vi "S4GUI_003.vi"(7 "Tab ObsEng":enum32{"Obs", "CCD modes", "Guider", "Eng"}(tab)) -> ()   [LabVIEW 2018] (continued)
        n4627 = call "Read WPROT.vi"("error in (no error)"=w10973, "Instrument in"=w10974) -> ("error out"=w10969:errorcluster, "Opt_Selector.lvclass"=w10972:refnum<class "Opt_Selector.lvclass">, "Instrument out"=w10965:refnum<class "Instrument.lvclass">)  [unwired: 7 in]
        n4628 = call-dynamic "Read State Machine.vi"("error in (no error)"=w10969, "Device in"=w10972) -> ("error out"=w10968:errorcluster, "State Machine.lvclass"=w10971:refnum<class "State Machine.lvclass">, "Device out"=w10967:refnum<class "Opt_Selector.lvclass">)  [unwired: 7 in]
        n4629 = call "Next State.vi"("error in (no error)"=w10968, "New_State"=1, "State Machine in"=w10971) -> ("error out"=w10956:errorcluster, "State Machine out"=w10958:refnum<class "State Machine.lvclass">)  [unwired: 7 in]
        n4630 = call-dynamic "Write Timer.vi"("error in (no error)"=w10956, "Timer"=u32 10, "State Machine in"=w10958) -> ("error out"=w10955:errorcluster, "State Machine out"=w10957:refnum<class "State Machine.lvclass">)  [unwired: 7 in]
        n4631 = call-dynamic "Write State Machine.vi"("error in (no error)"=w10955, "State Machine.lvclass"=w10957, "Device in"=w10967) -> ("error out"=w10964:errorcluster, "Device out"=w10966:refnum<class "Opt_Selector.lvclass">)  [unwired: 7 in]
        n4632 = call "Write WPROT.vi"("error in (no error)"=w10964, "Opt_Selector.lvclass"=w10966, "Instrument in"=w10965) -> ("error out"=w10961:errorcluster, "Instrument out"=w10963:refnum<class "Instrument.lvclass">)  [unwired: 7 in]
        n4633 = call "Write Instrument.lvclass.vi"("error in (no error)"=w10961, "Instrument.lvclass"=w10963, "S4ACS_GUI in"=w10962) -> ("error out"=w10960:errorcluster, "S4ACS_GUI out"=w10959:refnum<class "S4GUI.lvclass">)  [unwired: 7 in]
      }
      event "TARGET NAME WPROT": Value Change {
        n4634 = event-data() -> ()  [unwired: 1 in, 1 out]
        n4635 = call "Read Instrument.lvclass.vi"("error in (no error)"=w11004, "S4ACS_GUI in"=w11005) -> ("error out"=w11012:errorcluster, "Instrument.lvclass"=w11013:refnum<class "Instrument.lvclass">, "S4ACS_GUI out"=w11007:refnum<class "S4GUI.lvclass">)  [unwired: 7 in]
        n4636 = property on="TARGET NAME WPROT" class="Enum (strict)"() -> ("RingText.Text"=w11003:string)  [unwired: 2 in, 2 out]
        n4637 = Build Array(-1.0 ("element"), 0.0 ("element"), 22.5 ("element"), 45.0 ("element"), 67.5 ("element"), 90.0 ("element"), 112.5 ("element"), 135.0 ("element"), 157.5 ("element"), 180.0 ("element"), 202.5 ("element"), 225.0 ("element"), 247.5 ("element"), 270.0 ("element"), 292.5 ("element"), 315.0 ("element"), 337.5 ("element")) -> (w10995:dbl[])
        n4638 = call "Read WPROT.vi"("error in (no error)"=w11012, "Instrument in"=w11013) -> ("error out"=w11010:errorcluster, "Opt_Selector.lvclass"=w11011:refnum<class "Opt_Selector.lvclass">, "Instrument out"=w11009:refnum<class "Instrument.lvclass">)  [unwired: 7 in]
        n4639 = call "Write target name.vi"("error in (no error)"=w11010, "target name"=w11003, "Optics in"=w11011) -> ("error out"=w10991:errorcluster, "Optics out"=w10992:refnum<class "Opt_Selector.lvclass">)  [unwired: 7 in]
        n4640 = Index Array(array=w10995, index="TARGET NAME WPROT") -> (element=w10993:dbl)
        n4641 = call "Write target.vi"("error in (no error)"=w10991, "target"=w10993, "Optics in"=w10992) -> ("error out"=w10990:errorcluster, "Optics out"=w10989:refnum<class "Opt_Selector.lvclass">)  [unwired: 7 in]
        n4642 = call "Write WPROT.vi"("error in (no error)"=w10990, "Opt_Selector.lvclass"=w10989, "Instrument in"=w11009) -> ("error out"=w11006:errorcluster, "Instrument out"=w11008:refnum<class "Instrument.lvclass">)  [unwired: 7 in]
        n4643 = call "Write Instrument.lvclass.vi"("error in (no error)"=w11006, "Instrument.lvclass"=w11008, "S4ACS_GUI in"=w11007) -> ("error out"=w11002:errorcluster, "S4ACS_GUI out"=w10977:refnum<class "S4GUI.lvclass">)  [unwired: 7 in]
      }
      event "TARGET NAME WPSEL": Value Change {
        n4644 = event-data() -> ()  [unwired: 1 in, 1 out]
        n4645 = call "Read Instrument.lvclass.vi"("error in (no error)"=w11028, "S4ACS_GUI in"=w11029) -> ("error out"=w11036:errorcluster, "Instrument.lvclass"=w11037:refnum<class "Instrument.lvclass">, "S4ACS_GUI out"=w11031:refnum<class "S4GUI.lvclass">)  [unwired: 7 in]
        n4646 = property on="TARGET NAME WPSEL" class="Enum (strict)"() -> ("RingText.Text"=w11015:string)  [unwired: 2 in, 2 out]
        n4647 = Build Array(-1.0 ("element"), 80.0 ("element"), 0.0 ("element"), 160.0 ("element")) -> (w11022:dbl[])
        n4648 = call "Read WPSEL.vi"("error in (no error)"=w11036, "Instrument in"=w11037) -> ("error out"=w11034:errorcluster, "Opt_Selector.lvclass"=w11035:refnum<class "Opt_Selector.lvclass">, "Instrument out"=w11033:refnum<class "Instrument.lvclass">)  [unwired: 7 in]
        n4649 = call "Write target name.vi"("error in (no error)"=w11034, "target name"=w11015, "Optics in"=w11035) -> ("error out"=w11019:errorcluster, "Optics out"=w11020:refnum<class "Opt_Selector.lvclass">)  [unwired: 7 in]
        n4650 = Index Array(array=w11022, index="TARGET NAME WPSEL") -> (element=w11021:dbl)
        n4651 = call "Write target.vi"("error in (no error)"=w11019, "target"=w11021, "Optics in"=w11020) -> ("error out"=w11018:errorcluster, "Optics out"=w11017:refnum<class "Opt_Selector.lvclass">)  [unwired: 7 in]
        n4652 = call "Write WPSEL.vi"("error in (no error)"=w11018, "Opt_Selector.lvclass"=w11017, "Instrument in"=w11033) -> ("error out"=w11030:errorcluster, "Instrument out"=w11032:refnum<class "Instrument.lvclass">)  [unwired: 7 in]
        n4653 = call "Write Instrument.lvclass.vi"("error in (no error)"=w11030, "Instrument.lvclass"=w11032, "S4ACS_GUI in"=w11031) -> ("error out"=w11027:errorcluster, "S4ACS_GUI out"=w11014:refnum<class "S4GUI.lvclass">)  [unwired: 7 in]
      }
      event "Lambda Selector": Value Change {
        n4654 = event-data() -> ("NewVal"=w11039:u16)  [unwired: 1 in, 1 out]
        n4655 = call "Read Instrument.lvclass.vi"("error in (no error)"=w11070, "S4ACS_GUI in"=w11071) -> ("error out"=w11072:errorcluster, "Instrument.lvclass"=w11047:refnum<class "Instrument.lvclass">, "S4ACS_GUI out"=w11044:refnum<class "S4GUI.lvclass">)  [unwired: 7 in]
        n4656 = Build Array(80.0 ("element"), 0.0 ("element"), 160.0 ("element")) -> (w11065:dbl[])
        n4657 = property on="Lambda Selector" class="Ring (strict)"() -> ("RingText.Text"=w11045:string)  [unwired: 2 in, 2 out]
        n4658 = call "Read WPSEL.vi"("error in (no error)"=w11072, "Instrument in"=w11047) -> ("error out"=w11054:errorcluster, "Opt_Selector.lvclass"=w11053:refnum<class "Opt_Selector.lvclass">, "Instrument out"=w11046:refnum<class "Instrument.lvclass">)  [unwired: 7 in]
        n4659 = Index Array(array=w11065, index=w11039) -> (element=w11064:dbl)
        n4660 = call "Write target.vi"("error in (no error)"=w11054, "target"=w11064, "Optics in"=w11053) -> ("error out"=w11051:errorcluster, "Optics out"=w11052:refnum<class "Opt_Selector.lvclass">)  [unwired: 7 in]
        n4661 = case shown="\"OFF\", Default" w11045 {
          selector: w11045 -> [w11075 _ _]
          tunnel: [w11075 "ON" "ON"] -> w11056
          tunnel: [0.0 ("element") 30.0 ("element") 30.0 ("element")] -> w11055
          tunnel: [w11075 "L/2" "L/4"] -> w11048
          frame "OFF", Default {
            n4662 = property on="Calibrator Selector" class="Ring (strict)"("DisabledEnum"=T12."Disabled and Grayed Out" ("Disabled")) -> ()  [unwired: 2 in, 2 out]
          }
          frame "Lambda/2" {
            n4663 = property on="Calibrator Selector" class="Ring (strict)"("DisabledEnum"=T12."Enabled" ("Disabled")) -> ()  [unwired: 2 in, 2 out]
          }
          frame "Lambda/4" {
            n4664 = property on="Calibrator Selector" class="Ring (strict)"("DisabledEnum"=T12."Enabled" ("Disabled")) -> ()  [unwired: 2 in, 2 out]
          }
        }
        n4665 = call "Write target name.vi"("error in (no error)"=w11051, "target name"=w11048, "Optics in"=w11052) -> ("error out"=w11050:errorcluster, "Optics out"=w11049:refnum<class "Opt_Selector.lvclass">)  [unwired: 7 in]
        n4666 = call "Write WPSEL.vi"("error in (no error)"=w11050, "Opt_Selector.lvclass"=w11049, "Instrument in"=w11046) -> ("error out"=w11041:errorcluster, "Instrument out"=w11040:refnum<class "Instrument.lvclass">)  [unwired: 7 in]
        n4667 = call "Read ASEL.vi"("error in (no error)"=w11041, "Instrument in"=w11040) -> ("error out"=w11061:errorcluster, "Opt_Selector.lvclass"=w11059:refnum<class "Opt_Selector.lvclass">, "Instrument out"=w11043:refnum<class "Instrument.lvclass">)  [unwired: 7 in]
        n4668 = call "Write target name.vi"("error in (no error)"=w11061, "target name"=w11056, "Optics in"=w11059) -> ("error out"=w11062:errorcluster, "Optics out"=w11058:refnum<class "Opt_Selector.lvclass">)  [unwired: 7 in]
        n4669 = call "Write target.vi"("error in (no error)"=w11062, "target"=w11055, "Optics in"=w11058) -> ("error out"=w11063:errorcluster, "Optics out"=w11057:refnum<class "Opt_Selector.lvclass">)  [unwired: 7 in]
        n4670 = call "Write ASEL.vi"("error in (no error)"=w11063, "Opt_Selector.lvclass"=w11057, "Instrument in"=w11043) -> ("error out"=w11060:errorcluster, "Instrument out"=w11042:refnum<class "Instrument.lvclass">)  [unwired: 7 in]
        n4671 = call "Write Instrument.lvclass.vi"("error in (no error)"=w11060, "Instrument.lvclass"=w11042, "S4ACS_GUI in"=w11044) -> ("error out"=w11069:errorcluster, "S4ACS_GUI out"=w11038:refnum<class "S4GUI.lvclass">)  [unwired: 7 in]
      }
      event "Calibrator Selector": Value Change {
        n4672 = event-data() -> ()  [unwired: 1 in, 6 out]
        n4673 = call "Read Instrument.lvclass.vi"("error in (no error)"=w11104, "S4ACS_GUI in"=w11105) -> ("error out"=w11108:errorcluster, "Instrument.lvclass"=w11109:refnum<class "Instrument.lvclass">, "S4ACS_GUI out"=w11106:refnum<class "S4GUI.lvclass">)  [unwired: 7 in]
        n4674 = Build Array(0.0 ("element"), 72.0 ("element"), 144.0 ("element"), 216.0 ("element"), 288.0 ("element")) -> (w11099:dbl[])
        n4675 = call "Read CALW.vi"("error in (no error)"=w11108, "Instrument in"=w11109) -> ("error out"=w11097:errorcluster, "Opt_Selector.lvclass"=w11096:refnum<class "Opt_Selector.lvclass">, "Instrument out"=w11107:refnum<class "Instrument.lvclass">)  [unwired: 7 in]
        n4676 = Index Array(array=w11099, index="Calibrator Selector") -> (element=w11098:dbl)
        n4677 = call "Write target.vi"("error in (no error)"=w11097, "target"=w11098, "Optics in"=w11096) -> ("error out"=w11094:errorcluster, "Optics out"=w11095:refnum<class "Opt_Selector.lvclass">)  [unwired: 7 in]
        n4678 = property on="Calibrator Selector" class="Ring (strict)"() -> ("RingText.Text"=w11090:string)  [unwired: 2 in, 2 out]
        n4679 = case shown="\"POLARIZER\"" w11090 {
          selector: w11090 -> [_ w11111 w11112 w11113 w11114]
          tunnel: ["OFF" w11111 w11112 w11113 w11114] -> w11091
          frame "OFF", Default {
          }
          frame "POLARIZER" {
          }
          frame "DEPOLARIZER" {
          }
          frame "PINHOLE" {
          }
          frame "SHUTTER" {
          }
        }
        n4680 = call "Write target name.vi"("error in (no error)"=w11094, "target name"=w11091, "Optics in"=w11095) -> ("error out"=w11093:errorcluster, "Optics out"=w11092:refnum<class "Opt_Selector.lvclass">)  [unwired: 7 in]
        n4681 = call "Write CALW.vi"("error in (no error)"=w11093, "Opt_Selector.lvclass"=w11092, "Instrument in"=w11107) -> ("error out"=w11087:errorcluster, "Instrument out"=w11088:refnum<class "Instrument.lvclass">)  [unwired: 7 in]
        n4682 = call "Write Instrument.lvclass.vi"("error in (no error)"=w11087, "Instrument.lvclass"=w11088, "S4ACS_GUI in"=w11106) -> ("error out"=w11103:errorcluster, "S4ACS_GUI out"=w11086:refnum<class "S4GUI.lvclass">)  [unwired: 7 in]
      }
      event "TARGET NAME CALW": Value Change {
        # "aqui também"
        # "OV20230825: Valores da sequência original"
        n4683 = event-data() -> ()  [unwired: 1 in, 6 out]
        n4684 = call "Read Instrument.lvclass.vi"("error in (no error)"=w11131, "S4ACS_GUI in"=w11132) -> ("error out"=w11139:errorcluster, "Instrument.lvclass"=w11140:refnum<class "Instrument.lvclass">, "S4ACS_GUI out"=w11134:refnum<class "S4GUI.lvclass">)  [unwired: 7 in]
        n4685 = property on="TARGET NAME CALW" class="Enum (strict)"() -> ("RingText.Text"=w11115:string)  [unwired: 2 in, 2 out]
        n4686 = Build Array(-1.0 ("element"), 0.0 ("element"), 72.0 ("element"), 144.0 ("element"), 216.0 ("element"), 288.0 ("element")) -> (w11125:dbl[])
        n4687 = call "Read CALW.vi"("error in (no error)"=w11139, "Instrument in"=w11140) -> ("error out"=w11137:errorcluster, "Opt_Selector.lvclass"=w11138:refnum<class "Opt_Selector.lvclass">, "Instrument out"=w11136:refnum<class "Instrument.lvclass">)  [unwired: 7 in]
        n4688 = call "Write target name.vi"("error in (no error)"=w11137, "target name"=w11115, "Optics in"=w11138) -> ("error out"=w11122:errorcluster, "Optics out"=w11123:refnum<class "Opt_Selector.lvclass">)  [unwired: 7 in]
        n4689 = Index Array(array=w11125, index="TARGET NAME CALW") -> (element=w11124:dbl)
        n4690 = call "Write target.vi"("error in (no error)"=w11122, "target"=w11124, "Optics in"=w11123) -> ("error out"=w11121:errorcluster, "Optics out"=w11120:refnum<class "Opt_Selector.lvclass">)  [unwired: 7 in]
        n4691 = call "Write CALW.vi"("error in (no error)"=w11121, "Opt_Selector.lvclass"=w11120, "Instrument in"=w11136) -> ("error out"=w11133:errorcluster, "Instrument out"=w11135:refnum<class "Instrument.lvclass">)  [unwired: 7 in]
        n4692 = call "Write Instrument.lvclass.vi"("error in (no error)"=w11133, "Instrument.lvclass"=w11135, "S4ACS_GUI in"=w11134) -> ("error out"=w11130:errorcluster, "S4ACS_GUI out"=w11116:refnum<class "S4GUI.lvclass">)  [unwired: 7 in]
      }
      event "TARGET NAME ASEL": Value Change {
        n4693 = event-data() -> ()  [unwired: 1 in, 6 out]
        n4694 = call "Read Instrument.lvclass.vi"("error in (no error)"=w11154, "S4ACS_GUI in"=w11155) -> ("error out"=w11162:errorcluster, "Instrument.lvclass"=w11163:refnum<class "Instrument.lvclass">, "S4ACS_GUI out"=w11157:refnum<class "S4GUI.lvclass">)  [unwired: 7 in]
        n4695 = Build Array(-1.0 ("element"), 0.0 ("element"), 30.0 ("element")) -> (w11149:dbl[])
        n4696 = call "Read ASEL.vi"("error in (no error)"=w11162, "Instrument in"=w11163) -> ("error out"=w11160:errorcluster, "Opt_Selector.lvclass"=w11161:refnum<class "Opt_Selector.lvclass">, "Instrument out"=w11159:refnum<class "Instrument.lvclass">)  [unwired: 7 in]
        n4697 = property on="TARGET NAME ASEL" class="Enum (strict)"() -> ("RingText.Text"=w11143:string)  [unwired: 2 in, 2 out]
        n4698 = call "Write target name.vi"("error in (no error)"=w11160, "target name"=w11143, "Optics in"=w11161) -> ("error out"=w11146:errorcluster, "Optics out"=w11147:refnum<class "Opt_Selector.lvclass">)  [unwired: 7 in]
        n4699 = Index Array(array=w11149, index="TARGET NAME ASEL") -> (element=w11148:dbl)
        n4700 = call "Write target.vi"("error in (no error)"=w11146, "target"=w11148, "Optics in"=w11147) -> ("error out"=w11145:errorcluster, "Optics out"=w11144:refnum<class "Opt_Selector.lvclass">)  [unwired: 7 in]
        n4701 = call "Write ASEL.vi"("error in (no error)"=w11145, "Opt_Selector.lvclass"=w11144, "Instrument in"=w11159) -> ("error out"=w11156:errorcluster, "Instrument out"=w11158:refnum<class "Instrument.lvclass">)  [unwired: 7 in]
        n4702 = call "Write Instrument.lvclass.vi"("error in (no error)"=w11156, "Instrument.lvclass"=w11158, "S4ACS_GUI in"=w11157) -> ("error out"=w11153:errorcluster, "S4ACS_GUI out"=w11141:refnum<class "S4GUI.lvclass">)  [unwired: 7 in]
      }
      event "WPROT_stop": Value Change {
        n4703 = event-data() -> ()  [unwired: 1 in, 4 out]
        n4704 = call "Read Instrument.lvclass.vi"("error in (no error)"=w11182, "S4ACS_GUI in"=w11183) -> ("error out"=w11180:errorcluster, "Instrument.lvclass"=w11181:refnum<class "Instrument.lvclass">, "S4ACS_GUI out"=w11167:refnum<class "S4GUI.lvclass">)  [unwired: 7 in]
        n4705 = call "Read WPROT.vi"("error in (no error)"=w11180, "Instrument in"=w11181) -> ("error out"=w11176:errorcluster, "Opt_Selector.lvclass"=w11179:refnum<class "Opt_Selector.lvclass">, "Instrument out"=w11170:refnum<class "Instrument.lvclass">)  [unwired: 7 in]
        n4706 = call-dynamic "Read State Machine.vi"("error in (no error)"=w11176, "Device in"=w11179) -> ("error out"=w11175:errorcluster, "State Machine.lvclass"=w11178:refnum<class "State Machine.lvclass">, "Device out"=w11172:refnum<class "Opt_Selector.lvclass">)  [unwired: 7 in]
        n4707 = call "Next State.vi"("error in (no error)"=w11175, "New_State"=10, "State Machine in"=w11178) -> ("error out"=w11174:errorcluster, "State Machine out"=w11173:refnum<class "State Machine.lvclass">)  [unwired: 7 in]
        n4708 = call-dynamic "Write State Machine.vi"("error in (no error)"=w11174, "State Machine.lvclass"=w11173, "Device in"=w11172) -> ("error out"=w11169:errorcluster, "Device out"=w11171:refnum<class "Opt_Selector.lvclass">)  [unwired: 7 in]
        n4709 = call "Write WPROT.vi"("error in (no error)"=w11169, "Opt_Selector.lvclass"=w11171, "Instrument in"=w11170) -> ("error out"=w11166:errorcluster, "Instrument out"=w11168:refnum<class "Instrument.lvclass">)  [unwired: 7 in]
        n4710 = call "Write Instrument.lvclass.vi"("error in (no error)"=w11166, "Instrument.lvclass"=w11168, "S4ACS_GUI in"=w11167) -> ("error out"=w11165:errorcluster, "S4ACS_GUI out"=w11164:refnum<class "S4GUI.lvclass">)  [unwired: 7 in]
      }
      event "WPROT_init": Value Change {
        n4711 = event-data() -> ()  [unwired: 1 in, 4 out]
        n4712 = call "Read Instrument.lvclass.vi"("error in (no error)"=w11202, "S4ACS_GUI in"=w11203) -> ("error out"=w11200:errorcluster, "Instrument.lvclass"=w11201:refnum<class "Instrument.lvclass">, "S4ACS_GUI out"=w11187:refnum<class "S4GUI.lvclass">)  [unwired: 7 in]
        n4713 = call "Read WPROT.vi"("error in (no error)"=w11200, "Instrument in"=w11201) -> ("error out"=w11196:errorcluster, "Opt_Selector.lvclass"=w11199:refnum<class "Opt_Selector.lvclass">, "Instrument out"=w11190:refnum<class "Instrument.lvclass">)  [unwired: 7 in]
        n4714 = call-dynamic "Read State Machine.vi"("error in (no error)"=w11196, "Device in"=w11199) -> ("error out"=w11195:errorcluster, "State Machine.lvclass"=w11198:refnum<class "State Machine.lvclass">, "Device out"=w11192:refnum<class "Opt_Selector.lvclass">)  [unwired: 7 in]
        n4715 = call "Next State.vi"("error in (no error)"=w11195, "New_State"=30, "State Machine in"=w11198) -> ("error out"=w11194:errorcluster, "State Machine out"=w11193:refnum<class "State Machine.lvclass">)  [unwired: 7 in]
        n4716 = call-dynamic "Write State Machine.vi"("error in (no error)"=w11194, "State Machine.lvclass"=w11193, "Device in"=w11192) -> ("error out"=w11189:errorcluster, "Device out"=w11191:refnum<class "Opt_Selector.lvclass">)  [unwired: 7 in]
        n4717 = call "Write WPROT.vi"("error in (no error)"=w11189, "Opt_Selector.lvclass"=w11191, "Instrument in"=w11190) -> ("error out"=w11186:errorcluster, "Instrument out"=w11188:refnum<class "Instrument.lvclass">)  [unwired: 7 in]
        n4718 = call "Write Instrument.lvclass.vi"("error in (no error)"=w11186, "Instrument.lvclass"=w11188, "S4ACS_GUI in"=w11187) -> ("error out"=w11185:errorcluster, "S4ACS_GUI out"=w11184:refnum<class "S4GUI.lvclass">)  [unwired: 7 in]
      }
      event "WPSEL_target": Value Change {
        n4719 = event-data() -> ("NewVal"=w11213:dbl)  [unwired: 1 in, 3 out]
        n4720 = call "Read Instrument.lvclass.vi"("error in (no error)"=w11217, "S4ACS_GUI in"=w11218) -> ("error out"=w11215:errorcluster, "Instrument.lvclass"=w11216:refnum<class "Instrument.lvclass">, "S4ACS_GUI out"=w11207:refnum<class "S4GUI.lvclass">)  [unwired: 7 in]
        n4721 = call "Read WPSEL.vi"("error in (no error)"=w11215, "Instrument in"=w11216) -> ("error out"=w11212:errorcluster, "Opt_Selector.lvclass"=w11214:refnum<class "Opt_Selector.lvclass">, "Instrument out"=w11210:refnum<class "Instrument.lvclass">)  [unwired: 7 in]
        n4722 = call "Write target.vi"("error in (no error)"=w11212, "target"=w11213, "Optics in"=w11214) -> ("error out"=w11209:errorcluster, "Optics out"=w11211:refnum<class "Opt_Selector.lvclass">)  [unwired: 7 in]
        n4723 = call "Write WPSEL.vi"("error in (no error)"=w11209, "Opt_Selector.lvclass"=w11211, "Instrument in"=w11210) -> ("error out"=w11206:errorcluster, "Instrument out"=w11208:refnum<class "Instrument.lvclass">)  [unwired: 7 in]
        n4724 = call "Write Instrument.lvclass.vi"("error in (no error)"=w11206, "Instrument.lvclass"=w11208, "S4ACS_GUI in"=w11207) -> ("error out"=w11205:errorcluster, "S4ACS_GUI out"=w11204:refnum<class "S4GUI.lvclass">)  [unwired: 7 in]
      }
      event "WPSEL_set": Value Change {
        n4725 = event-data() -> ()  [unwired: 1 in, 4 out]
        n4726 = call "Read Instrument.lvclass.vi"("error in (no error)"=w11237, "S4ACS_GUI in"=w11238) -> ("error out"=w11235:errorcluster, "Instrument.lvclass"=w11236:refnum<class "Instrument.lvclass">, "S4ACS_GUI out"=w11223:refnum<class "S4GUI.lvclass">)  [unwired: 7 in]
        n4727 = call "Read WPSEL.vi"("error in (no error)"=w11235, "Instrument in"=w11236) -> ("error out"=w11232:errorcluster, "Opt_Selector.lvclass"=w11234:refnum<class "Opt_Selector.lvclass">, "Instrument out"=w11226:refnum<class "Instrument.lvclass">)  [unwired: 7 in]
        n4728 = call-dynamic "Read State Machine.vi"("error in (no error)"=w11232, "Device in"=w11234) -> ("error out"=w11231:errorcluster, "State Machine.lvclass"=w11220:refnum<class "State Machine.lvclass">, "Device out"=w11228:refnum<class "Opt_Selector.lvclass">)  [unwired: 7 in]
        n4729 = call "Next State.vi"("error in (no error)"=w11231, "New_State"=1, "State Machine in"=w11220) -> ("error out"=w11230:errorcluster, "State Machine out"=w11229:refnum<class "State Machine.lvclass">)  [unwired: 7 in]
        n4730 = call-dynamic "Write State Machine.vi"("error in (no error)"=w11230, "State Machine.lvclass"=w11229, "Device in"=w11228) -> ("error out"=w11225:errorcluster, "Device out"=w11227:refnum<class "Opt_Selector.lvclass">)  [unwired: 7 in]
        n4731 = call "Write WPSEL.vi"("error in (no error)"=w11225, "Opt_Selector.lvclass"=w11227, "Instrument in"=w11226) -> ("error out"=w11222:errorcluster, "Instrument out"=w11224:refnum<class "Instrument.lvclass">)  [unwired: 7 in]
        n4732 = call "Write Instrument.lvclass.vi"("error in (no error)"=w11222, "Instrument.lvclass"=w11224, "S4ACS_GUI in"=w11223) -> ("error out"=w11221:errorcluster, "S4ACS_GUI out"=w11219:refnum<class "S4GUI.lvclass">)  [unwired: 7 in]
      }
      event "Set Waveplate": Value Change {
        # "OV20230825: Sequência de\nvalores originais."
        # "Garantir que, quando em POLARIMETRIA, pelo menos WP1 esteja selecionado."
        n4733 = event-data() -> ()  [unwired: 1 in, 4 out]
        n4734 = local read "Lambda Selector"() -> (w11342:u16)
        n4735 = property on="Calibrator Selector" class="Ring (strict)"() -> ("RingText.Text"=w11323:string)  [unwired: 2 in, 2 out]
        n4736 = call "Read Instrument.lvclass.vi"("error in (no error)"=w11322, "S4ACS_GUI in"=w11321) -> ("error out"=w11340:errorcluster, "Instrument.lvclass"=w11341:refnum<class "Instrument.lvclass">, "S4ACS_GUI out"=w11338:refnum<class "S4GUI.lvclass">)  [unwired: 7 in]
        n4737 = Build Array(0.0 ("element"), 72.0 ("element"), 144.0 ("element"), 216.0 ("element"), 288.0 ("element")) -> (w11334:dbl[])
        n4738 = local read "Calibrator Selector"() -> (w11324:u16)
        n4739 = Build Array(80.0 ("element"), 0.0 ("element"), 160.0 ("element")) -> (w11368:dbl[])
        n4740 = property on="Lambda Selector" class="Ring (strict)"() -> ("RingText.Text"=w11343:string)  [unwired: 2 in, 2 out]
        n4741 = call "Read CALW.vi"("error in (no error)"=w11340, "Instrument in"=w11341) -> ("error out"=w11332:errorcluster, "Opt_Selector.lvclass"=w11331:refnum<class "Opt_Selector.lvclass">, "Instrument out"=w11339:refnum<class "Instrument.lvclass">)  [unwired: 7 in]
        n4742 = Index Array(array=w11334, index=w11324) -> (element=w11333:dbl)
        n4743 = Index Array(array=w11368, index=w11342) -> (element=w11367:dbl)
        n4744 = call "Write target.vi"("error in (no error)"=w11332, "target"=w11333, "Optics in"=w11331) -> ("error out"=w11329:errorcluster, "Optics out"=w11330:refnum<class "Opt_Selector.lvclass">)  [unwired: 7 in]
        n4745 = case shown="\"OFF\", Default" w11323 {
          tunnel: ["OFF" w11597 "PINHOLE" "SHUTTER" w11602] -> w11241
          frame "OFF", Default {
          }
          frame "POLARIZER" {
            n4746 = disable-structure shown="Enabled" {
              disable-tunnel: ["POLARIZER" "DEPOLARIZER"] -> w11597
              frame Enabled {
              }
              frame Disabled {
                # "OV20230426: Montagem do CALW\nestá com POL e DEPOL invertidos"
              }
            }
          }
          frame "PINHOLE" {
          }
          frame "SHUTTER" {
          }
          frame "DEPOLARIZER" {
            n4747 = disable-structure shown="Enabled" {
              disable-tunnel: ["POLARIZER" "DEPOLARIZER"] -> w11602
              frame Disabled {
                # "OV20230426: Montagem do CALW\nestá com POL e DEPOL invertidos"
              }
              frame Enabled {
              }
            }
          }
        }
        n4748 = case shown="\"OFF\", Default" w11343 {
          tunnel: [w11605 "ON" "ON"] -> w11254
          tunnel: [w11606 w11607 w11610] -> w11359
          tunnel: [w11605 "L/2" "L/4"] -> w11239
          tunnel: [w11606 w11607 w11610] -> w11243
          frame "OFF", Default {
            w11605 = "OFF"
            w11606 = 0.0 ("element")
            n4749 = property on="Lambda Selector" class="Ring (strict)"("RingText.Text"=w11605) -> ()  [unwired: 2 in, 2 out]
          }
          frame "Lambda/2" {
            w11607 = 30.0 ("element")
          }
          frame "Lambda/4" {
            w11610 = 30.0 ("element")
          }
        }
        n4750 = call "Write target name.vi"("error in (no error)"=w11329, "target name"=w11241, "Optics in"=w11330) -> ("error out"=w11328:errorcluster, "Optics out"=w11327:refnum<class "Opt_Selector.lvclass">)  [unwired: 7 in]
        n4751 = call "Write CALW.vi"("error in (no error)"=w11328, "Opt_Selector.lvclass"=w11327, "Instrument in"=w11339) -> ("error out"=w11325:errorcluster, "Instrument out"=w11326:refnum<class "Instrument.lvclass">)  [unwired: 7 in]
        n4752 = Equal To 0?(x=w11243) -> (x = 0?=w11244:bool)
        n4753 = call "Write Instrument.lvclass.vi"("error in (no error)"=w11325, "Instrument.lvclass"=w11326, "S4ACS_GUI in"=w11338) -> ("error out"=w11319:errorcluster, "S4ACS_GUI out"=w11320:refnum<class "S4GUI.lvclass">)  [unwired: 7 in]
        n4754 = call "Read Instrument.lvclass.vi"("error in (no error)"=w11319, "S4ACS_GUI in"=w11320) -> ("error out"=w11372:errorcluster, "Instrument.lvclass"=w11352:refnum<class "Instrument.lvclass">, "S4ACS_GUI out"=w11350:refnum<class "S4GUI.lvclass">)  [unwired: 7 in]
        n4755 = call "Read WPSEL.vi"("error in (no error)"=w11372, "Instrument in"=w11352) -> ("error out"=w11358:errorcluster, "Opt_Selector.lvclass"=w11357:refnum<class "Opt_Selector.lvclass">, "Instrument out"=w11351:refnum<class "Instrument.lvclass">)  [unwired: 7 in]
        n4756 = call "Write target.vi"("error in (no error)"=w11358, "target"=w11367, "Optics in"=w11357) -> ("error out"=w11355:errorcluster, "Optics out"=w11356:refnum<class "Opt_Selector.lvclass">)  [unwired: 7 in]
        n4757 = call "Write target name.vi"("error in (no error)"=w11355, "target name"=w11239, "Optics in"=w11356) -> ("error out"=w11354:errorcluster, "Optics out"=w11353:refnum<class "Opt_Selector.lvclass">)  [unwired: 7 in]
        n4758 = call "Write WPSEL.vi"("error in (no error)"=w11354, "Opt_Selector.lvclass"=w11353, "Instrument in"=w11351) -> ("error out"=w11347:errorcluster, "Instrument out"=w11346:refnum<class "Instrument.lvclass">)  [unwired: 7 in]
        n4759 = call "Read ASEL.vi"("error in (no error)"=w11347, "Instrument in"=w11346) -> ("error out"=w11364:errorcluster, "Opt_Selector.lvclass"=w11362:refnum<class "Opt_Selector.lvclass">, "Instrument out"=w11349:refnum<class "Instrument.lvclass">)  [unwired: 7 in]
        n4760 = call "Write target name.vi"("error in (no error)"=w11364, "target name"=w11254, "Optics in"=w11362) -> ("error out"=w11365:errorcluster, "Optics out"=w11361:refnum<class "Opt_Selector.lvclass">)  [unwired: 7 in]
        n4761 = Select(t="OFF", s=w11244, f=w11241) -> (s? t:f=w11242:string)
        n4762 = call "Write target.vi"("error in (no error)"=w11365, "target"=w11359, "Optics in"=w11361) -> ("error out"=w11366:errorcluster, "Optics out"=w11360:refnum<class "Opt_Selector.lvclass">)  [unwired: 7 in]
        n4763 = call "Write ASEL.vi"("error in (no error)"=w11366, "Opt_Selector.lvclass"=w11360, "Instrument in"=w11349) -> ("error out"=w11363:errorcluster, "Instrument out"=w11348:refnum<class "Instrument.lvclass">)  [unwired: 7 in]
        n4764 = call "Write Instrument.lvclass.vi"("error in (no error)"=w11363, "Instrument.lvclass"=w11348, "S4ACS_GUI in"=w11350) -> ("error out"=w11344:errorcluster, "S4ACS_GUI out"=w11345:refnum<class "S4GUI.lvclass">)  [unwired: 7 in]
        n4765 = call "Read Instrument.lvclass.vi"("error in (no error)"=w11344, "S4ACS_GUI in"=w11345) -> ("error out"=w11413:errorcluster, "Instrument.lvclass"=w11414:refnum<class "Instrument.lvclass">, "S4ACS_GUI out"=w11260:refnum<class "S4GUI.lvclass">)  [unwired: 7 in]
        n4766 = call "Read WPSEL.vi"("error in (no error)"=w11413, "Instrument in"=w11414) -> ("error out"=w11410:errorcluster, "Opt_Selector.lvclass"=w11412:refnum<class "Opt_Selector.lvclass">, "Instrument out"=w11404:refnum<class "Instrument.lvclass">)  [unwired: 7 in]
        n4767 = call-dynamic "Read State Machine.vi"("error in (no error)"=w11410, "Device in"=w11412) -> ("error out"=w11409:errorcluster, "State Machine.lvclass"=w11402:refnum<class "State Machine.lvclass">, "Device out"=w11406:refnum<class "Opt_Selector.lvclass">)  [unwired: 7 in]
        n4768 = call "Next State.vi"("error in (no error)"=w11409, "New_State"=1, "State Machine in"=w11402) -> ("error out"=w11408:errorcluster, "State Machine out"=w11407:refnum<class "State Machine.lvclass">)  [unwired: 7 in]
        n4769 = call-dynamic "Write State Machine.vi"("error in (no error)"=w11408, "State Machine.lvclass"=w11407, "Device in"=w11406) -> ("error out"=w11403:errorcluster, "Device out"=w11405:refnum<class "Opt_Selector.lvclass">)  [unwired: 7 in]
        n4770 = call "Write WPSEL.vi"("error in (no error)"=w11403, "Opt_Selector.lvclass"=w11405, "Instrument in"=w11404) -> ("error out"=w11394:errorcluster, "Instrument out"=w11393:refnum<class "Instrument.lvclass">)  [unwired: 7 in]
        n4771 = call "Read ASEL.vi"("error in (no error)"=w11394, "Instrument in"=w11393) -> ("error out"=w11400:errorcluster, "Opt_Selector.lvclass"=w11391:refnum<class "Opt_Selector.lvclass">, "Instrument out"=w11392:refnum<class "Instrument.lvclass">)  [unwired: 7 in]
        n4772 = call-dynamic "Read State Machine.vi"("error in (no error)"=w11400, "Device in"=w11391) -> ("error out"=w11399:errorcluster, "State Machine.lvclass"=w11395:refnum<class "State Machine.lvclass">, "Device out"=w11390:refnum<class "Opt_Selector.lvclass">)  [unwired: 7 in]
        n4773 = call "Next State.vi"("error in (no error)"=w11399, "New_State"=1, "State Machine in"=w11395) -> ("error out"=w11398:errorcluster, "State Machine out"=w11397:refnum<class "State Machine.lvclass">)  [unwired: 7 in]
        n4774 = call-dynamic "Write State Machine.vi"("error in (no error)"=w11398, "State Machine.lvclass"=w11397, "Device in"=w11390) -> ("error out"=w11396:errorcluster, "Device out"=w11389:refnum<class "Opt_Selector.lvclass">)  [unwired: 7 in]
        n4775 = Concatenate Strings("SET WAVEPLATE:  WPSEL=" ("string"), w11239, " CALW=" ("string"), w11242) -> (w11252:string)
        n4776 = call "Write ASEL.vi"("error in (no error)"=w11396, "Opt_Selector.lvclass"=w11389, "Instrument in"=w11392) -> ("error out"=w11376:errorcluster, "Instrument out"=w11378:refnum<class "Instrument.lvclass">)  [unwired: 7 in]
        n4777 = call "Read CALW.vi"("error in (no error)"=w11376, "Instrument in"=w11378) -> ("error out"=w11386:errorcluster, "Opt_Selector.lvclass"=w11388:refnum<class "Opt_Selector.lvclass">, "Instrument out"=w11377:refnum<class "Instrument.lvclass">)  [unwired: 7 in]
        n4778 = call-dynamic "Read State Machine.vi"("error in (no error)"=w11386, "Device in"=w11388) -> ("error out"=w11385:errorcluster, "State Machine.lvclass"=w11379:refnum<class "State Machine.lvclass">, "Device out"=w11382:refnum<class "Opt_Selector.lvclass">)  [unwired: 7 in]
        n4779 = call "Next State.vi"("error in (no error)"=w11385, "New_State"=1, "State Machine in"=w11379) -> ("error out"=w11384:errorcluster, "State Machine out"=w11383:refnum<class "State Machine.lvclass">)  [unwired: 7 in]
        n4780 = call-dynamic "Write State Machine.vi"("error in (no error)"=w11384, "State Machine.lvclass"=w11383, "Device in"=w11382) -> ("error out"=w11380:errorcluster, "Device out"=w11381:refnum<class "Opt_Selector.lvclass">)  [unwired: 7 in]
        n4781 = property on="Lambda Selector" class="Ring (strict)"() -> ("RingText.Text"=w11375:string)  [unwired: 2 in, 2 out]
        n4782 = call "Write CALW.vi"("error in (no error)"=w11380, "Opt_Selector.lvclass"=w11381, "Instrument in"=w11377) -> ("error out"=w11259:errorcluster, "Instrument out"=w11374:refnum<class "Instrument.lvclass">)  [unwired: 7 in]
        n4783 = call-dynamic "Read mode EXPOSE.vi"("error in (no error)"=w11259, "S4GUI in"=w11260) -> ("error out"=w11258:errorcluster, "mode EXPOSE"=w11256:bool, "S4GUI out"=w11257:refnum<class "S4GUI.lvclass">)  [unwired: 7 in]
        n4784 = call-dynamic "Read sync.vi"("error in (no error)"=w11258, "S4ACS_GUI in"=w11257) -> ("error out"=w11276:errorcluster, "sync"=w11275:bool, "S4ACS_GUI out"=w11277:refnum<class "S4GUI.lvclass">)  [unwired: 7 in]
        n4785 = case shown="\"OFF\"" w11375 {
          selector: w11375 -> [w11622 _]
          tunnel: w11374 -> [w11626 w11644]
          tunnel: [w11625 w11644] -> w11373
          tunnel: [w11618 w11643] -> w11293
          tunnel: w11276 -> [w11624 w11643]
          tunnel: [w11615 w11639] -> w11288
          tunnel: w11275 -> [w11614 _]
          tunnel: w11256 -> [w11613 w11642]
          frame "OFF" {
            w11616 = u16 0 items=["OFF", "POLARIZER", "PINHOLE", "SHUTTER", "DEPOLARIZER"] ("Calibrator Selector 2")
            n4786 = call "Read CALW.vi"("error in (no error)"=w11624, "Instrument in"=w11626) -> ("error out"=w11629:errorcluster, "Opt_Selector.lvclass"=w11631:refnum<class "Opt_Selector.lvclass">, "Instrument out"=w11630:refnum<class "Instrument.lvclass">)  [unwired: 7 in]
            n4787 = call "Write target.vi"("error in (no error)"=w11629, "target"=0.0, "Optics in"=w11631) -> ("error out"=w11628:errorcluster, "Optics out"=w11632:refnum<class "Opt_Selector.lvclass">)  [unwired: 7 in]
            n4788 = call "Write target name.vi"("error in (no error)"=w11628, "target name"=w11622, "Optics in"=w11632) -> ("error out"=w11627:errorcluster, "Optics out"=w11633:refnum<class "Opt_Selector.lvclass">)  [unwired: 7 in]
            n4789 = call "Write CALW.vi"("error in (no error)"=w11627, "Opt_Selector.lvclass"=w11633, "Instrument in"=w11630) -> ("error out"=w11617:errorcluster, "Instrument out"=w11625:refnum<class "Instrument.lvclass">)  [unwired: 7 in]
            n4790 = property on="Calibrator Selector" class="Ring (strict)"(error in=w11617, "Value"=w11616, "DisabledEnum"=T12."Disabled and Grayed Out" ("Disabled")) -> (error out=w11619:errorcluster)  [unwired: 1 in, 1 out]
            n4791 = property on="Calibrator Selector" class="Ring (strict)"(error in=w11619, "RingText.Text"="OFF" ("Ring Text.Text")) -> (error out=w11618:errorcluster)  [unwired: 1 in, 1 out]
            n4792 = case shown="True" w11614 {
              tunnel: [u8 0 ("SHUTTER_MODE") w11636] -> w11615
              tunnel: w11613 -> [_ w11635]
              frame False {
                # "Fotom. & Async"
                # "Internal"
              }
              frame True {
                # "Ext. Start"
                # "Internal"
                # "Fotom. Sync. SEM exp mode"
                # "Fotom. Sync. COM exp mode"
                n4793 = Select(t=u8 0, s=w11635, f=u8 6 ("SHUTTER_MODE")) -> (s? t:f=w11636:u8)
              }
            }
          }
          frame Default {
            # "Polar. COM exp mode"
            # "Internal"
            # "Polar. SEM exp mode"
            # "Ext. Start"
            n4794 = Select(t=u8 0, s=w11642, f=u8 6 ("SHUTTER_MODE")) -> (s? t:f=w11639:u8)
          }
        }
        n4795 = call "Write Instrument.lvclass.vi"("error in (no error)"=w11293, "Instrument.lvclass"=w11373, "S4ACS_GUI in"=w11277) -> ("error out"=w11292:errorcluster, "S4ACS_GUI out"=w11281:refnum<class "S4GUI.lvclass">)  [unwired: 7 in]
        n4796 = call-dynamic "Read AcquisitionC.vi"("error in (no error)"=w11292, "S4ACS_GUI in"=w11281) -> ("error out"=w11303:errorcluster, "Acquisition.lvclass"=w11302:refnum<class "Acquisition.lvclass">)  [unwired: 7 in, 1 out]
        n4797 = call-dynamic "Read AcquisitionA.vi"("error in (no error)"=w11292, "S4ACS_GUI in"=w11281) -> ("error out"=w11306:errorcluster, "Acquisition.lvclass"=w11307:refnum<class "Acquisition.lvclass">)  [unwired: 7 in, 1 out]
        n4798 = call "Read AcquisitionB.vi"("error in (no error)"=w11292, "S4ACS_GUI in"=w11281) -> ("error out"=w11304:errorcluster, "Acquisition.lvclass"=w11305:refnum<class "Acquisition.lvclass">)  [unwired: 7 in, 1 out]
        n4799 = call-dynamic "Read AcquisitionD.vi"("error in (no error)"=w11292, "S4ACS_GUI in"=w11281) -> ("error out"=w11300:errorcluster, "Acquisition.lvclass"=w11301:refnum<class "Acquisition.lvclass">)  [unwired: 7 in, 1 out]
        n4800 = call "Read connection.vi"("error in (no error)"=w11303, "Server in"=w11302) -> ("error out"=w11309:errorcluster, "connection"=w11308:bool, "Server out"=w11310:refnum<class "Acquisition.lvclass">)  [unwired: 7 in]
        n4801 = call "Read connection.vi"("error in (no error)"=w11304, "Server in"=w11305) -> ("error out"=w11312:errorcluster, "connection"=w11311:bool, "Server out"=w11313:refnum<class "Acquisition.lvclass">)  [unwired: 7 in]
        n4802 = call "Read connection.vi"("error in (no error)"=w11300, "Server in"=w11301) -> ("error out"=w11289:errorcluster, "connection"=w11290:bool, "Server out"=w11291:refnum<class "Acquisition.lvclass">)  [unwired: 7 in]
        n4803 = call "Read connection.vi"("error in (no error)"=w11306, "Server in"=w11307) -> ("error out"=w11315:errorcluster, "connection"=w11314:bool, "Server out"=w11316:refnum<class "Acquisition.lvclass">)  [unwired: 7 in]
        n4804 = case shown="True" w11308 {
          tunnel: w11310 -> [w11480 w11485]
          tunnel: w11309 -> [w11479 w11484]
          tunnel: [w11480 w11483] -> w11295
          tunnel: [w11479 w11482] -> w11294
          tunnel: w11288 -> [_ w11481]
          frame False {
          }
          frame True {
            # "nome do arquivo .cfg"
            # "seção no arquivo .cfg"
            n4805 = call-dynamic "Read Channel.vi"("error in (no error)"=w11484, "Acquisition in"=w11485) -> ("error out"=w11489:errorcluster, "Channel.lvclass"=w11488:refnum<class "Channel.lvclass">, "Acquisition out"=w11487:refnum<class "Acquisition.lvclass">)  [unwired: 7 in]
            n4806 = call-dynamic "Read Interface.vi"("error in (no error)"=w11489, "Channel in"=w11488) -> ("error out"=w11496:errorcluster, "Interface.lvclass"=w11497:refnum<class "Interface.lvclass">, "Channel out"=w11486:refnum<class "Channel.lvclass">)  [unwired: 7 in]
            n4807 = call-dynamic "Get CCD_Config.vi"("error in (no error)"=w11496, "Interface in"=w11497) -> ("error out"=w11494:errorcluster, "output cluster"=w11493:T31, "Interface out"=w11498:refnum<class "Interface.lvclass">)  [unwired: 7 in]
            n4808 = Bundle By Name(cluster=w11493, "TRIGGER_MODE"=w11481) -> (w11495:T31)
            n4809 = call-dynamic "Set CCD_Config.vi"("error in (no error)"=w11494, "input cluster"=w11495, "Interface in"=w11498) -> ("error out"=w11492:errorcluster, "Interface out"=w11499:refnum<class "Interface.lvclass">)  [unwired: 7 in]
            n4810 = Flatten To String(anything=w11495, error in (no error)=w11492) -> (data string=w11490:string, error out=w11491:errorcluster)  [unwired: 2 in, 1 out]
            n4811 = call "Write flatted cluster.vi"("error in (no error)"=w11491, "flatted cluster"=w11490, "Interface in"=w11499) -> ("error out"=w11501:errorcluster, "Interface out"=w11500:refnum<class "Interface.lvclass">)  [unwired: 7 in]
            n4812 = call-dynamic "Write Interface.vi"("error in (no error)"=w11501, "Interface.lvclass"=w11500, "Channel in"=w11486) -> ("error out"=w11507:errorcluster, "Channel out"=w11508:refnum<class "Channel.lvclass">)  [unwired: 7 in]
            n4813 = call "Write section_name.vi"("error in (no error)"=w11507, "section_name"="CCD_ACS3", "Channel in"=w11508) -> ("error out"=w11505:errorcluster, "Channel out"=w11511:refnum<class "Channel.lvclass">)  [unwired: 7 in]
            n4814 = call-dynamic "save config.vi"("error in (no error)"=w11505, "file config"="lastsaved.cfg", "Channel in"=w11511) -> ("error out"=w11506:errorcluster, "Channel out"=w11512:refnum<class "Channel.lvclass">)  [unwired: 7 in]
            n4815 = call-dynamic "Read State Machine.vi"("error in (no error)"=w11506, "Device in"=w11512) -> ("error out"=w11502:errorcluster, "State Machine.lvclass"=w11514:refnum<class "State Machine.lvclass">, "Device out"=w11513:refnum<class "Channel.lvclass">)  [unwired: 7 in]
            n4816 = call-dynamic "Write State.vi"("error in (no error)"=w11502, "State"=60, "State Machine in"=w11514) -> ("error out"=w11503:errorcluster, "State Machine out"=w11515:refnum<class "State Machine.lvclass">)  [unwired: 7 in]
            n4817 = call-dynamic "Write State Machine.vi"("error in (no error)"=w11503, "State Machine.lvclass"=w11515, "Device in"=w11513) -> ("error out"=w11517:errorcluster, "Device out"=w11516:refnum<class "Channel.lvclass">)  [unwired: 7 in]
            n4818 = call-dynamic "Write Channel.vi"("error in (no error)"=w11517, "Channel.lvclass"=w11516, "Acquisition in"=w11487) -> ("error out"=w11482:errorcluster, "Acquisition out"=w11483:refnum<class "Acquisition.lvclass">)  [unwired: 7 in]
          }
        }
        n4819 = case shown="True" w11290 {
          tunnel: w11291 -> [w11441 w11446]
          tunnel: w11289 -> [w11440 w11445]
          tunnel: w11288 -> [_ w11444]
          tunnel: [w11441 w11443] -> w11287
          tunnel: [w11440 w11442] -> w11286
          frame False {
          }
          frame True {
            # "nome do arquivo .cfg"
            # "seção no arquivo .cfg"
            n4820 = call-dynamic "Read Channel.vi"("error in (no error)"=w11445, "Acquisition in"=w11446) -> ("error out"=w11475:errorcluster, "Channel.lvclass"=w11476:refnum<class "Channel.lvclass">, "Acquisition out"=w11477:refnum<class "Acquisition.lvclass">)  [unwired: 7 in]
            n4821 = call-dynamic "Read Interface.vi"("error in (no error)"=w11475, "Channel in"=w11476) -> ("error out"=w11468:errorcluster, "Interface.lvclass"=w11467:refnum<class "Interface.lvclass">, "Channel out"=w11478:refnum<class "Channel.lvclass">)  [unwired: 7 in]
            n4822 = call-dynamic "Get CCD_Config.vi"("error in (no error)"=w11468, "Interface in"=w11467) -> ("error out"=w11470:errorcluster, "output cluster"=w11471:T31, "Interface out"=w11466:refnum<class "Interface.lvclass">)  [unwired: 7 in]
            n4823 = Bundle By Name(cluster=w11471, "TRIGGER_MODE"=w11444) -> (w11469:T31)
            n4824 = call-dynamic "Set CCD_Config.vi"("error in (no error)"=w11470, "input cluster"=w11469, "Interface in"=w11466) -> ("error out"=w11472:errorcluster, "Interface out"=w11465:refnum<class "Interface.lvclass">)  [unwired: 7 in]
            n4825 = Flatten To String(anything=w11469, error in (no error)=w11472) -> (data string=w11474:string, error out=w11473:errorcluster)  [unwired: 2 in, 1 out]
            n4826 = call "Write flatted cluster.vi"("error in (no error)"=w11473, "flatted cluster"=w11474, "Interface in"=w11465) -> ("error out"=w11463:errorcluster, "Interface out"=w11464:refnum<class "Interface.lvclass">)  [unwired: 7 in]
            n4827 = call-dynamic "Write Interface.vi"("error in (no error)"=w11463, "Interface.lvclass"=w11464, "Channel in"=w11478) -> ("error out"=w11457:errorcluster, "Channel out"=w11456:refnum<class "Channel.lvclass">)  [unwired: 7 in]
            n4828 = call "Write section_name.vi"("error in (no error)"=w11457, "section_name"="CCD_ACS4", "Channel in"=w11456) -> ("error out"=w11459:errorcluster, "Channel out"=w11453:refnum<class "Channel.lvclass">)  [unwired: 7 in]
            n4829 = call-dynamic "save config.vi"("error in (no error)"=w11459, "file config"="lastsaved.cfg", "Channel in"=w11453) -> ("error out"=w11458:errorcluster, "Channel out"=w11452:refnum<class "Channel.lvclass">)  [unwired: 7 in]
            n4830 = call-dynamic "Read State Machine.vi"("error in (no error)"=w11458, "Device in"=w11452) -> ("error out"=w11462:errorcluster, "State Machine.lvclass"=w11450:refnum<class "State Machine.lvclass">, "Device out"=w11451:refnum<class "Channel.lvclass">)  [unwired: 7 in]
            n4831 = call-dynamic "Write State.vi"("error in (no error)"=w11462, "State"=60, "State Machine in"=w11450) -> ("error out"=w11461:errorcluster, "State Machine out"=w11449:refnum<class "State Machine.lvclass">)  [unwired: 7 in]
            n4832 = call-dynamic "Write State Machine.vi"("error in (no error)"=w11461, "State Machine.lvclass"=w11449, "Device in"=w11451) -> ("error out"=w11447:errorcluster, "Device out"=w11448:refnum<class "Channel.lvclass">)  [unwired: 7 in]
            n4833 = call-dynamic "Write Channel.vi"("error in (no error)"=w11447, "Channel.lvclass"=w11448, "Acquisition in"=w11477) -> ("error out"=w11442:errorcluster, "Acquisition out"=w11443:refnum<class "Acquisition.lvclass">)  [unwired: 7 in]
          }
        }
        n4834 = case shown="True" w11311 {
          tunnel: w11313 -> [w11519 w11524]
          tunnel: w11312 -> [w11518 w11523]
          tunnel: [w11519 w11522] -> w11297
          tunnel: [w11518 w11521] -> w11296
          tunnel: w11288 -> [_ w11520]
          frame False {
          }
          frame True {
            # "nome do arquivo .cfg"
            # "seção no arquivo .cfg"
            n4835 = call-dynamic "Read Channel.vi"("error in (no error)"=w11523, "Acquisition in"=w11524) -> ("error out"=w11528:errorcluster, "Channel.lvclass"=w11527:refnum<class "Channel.lvclass">, "Acquisition out"=w11526:refnum<class "Acquisition.lvclass">)  [unwired: 7 in]
            n4836 = call-dynamic "Read Interface.vi"("error in (no error)"=w11528, "Channel in"=w11527) -> ("error out"=w11535:errorcluster, "Interface.lvclass"=w11536:refnum<class "Interface.lvclass">, "Channel out"=w11525:refnum<class "Channel.lvclass">)  [unwired: 7 in]
            n4837 = call-dynamic "Get CCD_Config.vi"("error in (no error)"=w11535, "Interface in"=w11536) -> ("error out"=w11533:errorcluster, "output cluster"=w11532:T31, "Interface out"=w11537:refnum<class "Interface.lvclass">)  [unwired: 7 in]
            n4838 = Bundle By Name(cluster=w11532, "TRIGGER_MODE"=w11520) -> (w11534:T31)
            n4839 = call-dynamic "Set CCD_Config.vi"("error in (no error)"=w11533, "input cluster"=w11534, "Interface in"=w11537) -> ("error out"=w11531:errorcluster, "Interface out"=w11538:refnum<class "Interface.lvclass">)  [unwired: 7 in]
            n4840 = Flatten To String(anything=w11534, error in (no error)=w11531) -> (data string=w11529:string, error out=w11530:errorcluster)  [unwired: 2 in, 1 out]
            n4841 = call "Write flatted cluster.vi"("error in (no error)"=w11530, "flatted cluster"=w11529, "Interface in"=w11538) -> ("error out"=w11540:errorcluster, "Interface out"=w11539:refnum<class "Interface.lvclass">)  [unwired: 7 in]
            n4842 = call-dynamic "Write Interface.vi"("error in (no error)"=w11540, "Interface.lvclass"=w11539, "Channel in"=w11525) -> ("error out"=w11546:errorcluster, "Channel out"=w11547:refnum<class "Channel.lvclass">)  [unwired: 7 in]
            n4843 = call "Write section_name.vi"("error in (no error)"=w11546, "section_name"="CCD_ACS2", "Channel in"=w11547) -> ("error out"=w11544:errorcluster, "Channel out"=w11550:refnum<class "Channel.lvclass">)  [unwired: 7 in]
            n4844 = call-dynamic "save config.vi"("error in (no error)"=w11544, "file config"="lastsaved.cfg", "Channel in"=w11550) -> ("error out"=w11545:errorcluster, "Channel out"=w11551:refnum<class "Channel.lvclass">)  [unwired: 7 in]
            n4845 = call-dynamic "Read State Machine.vi"("error in (no error)"=w11545, "Device in"=w11551) -> ("error out"=w11541:errorcluster, "State Machine.lvclass"=w11553:refnum<class "State Machine.lvclass">, "Device out"=w11552:refnum<class "Channel.lvclass">)  [unwired: 7 in]
            n4846 = call-dynamic "Write State.vi"("error in (no error)"=w11541, "State"=60, "State Machine in"=w11553) -> ("error out"=w11542:errorcluster, "State Machine out"=w11554:refnum<class "State Machine.lvclass">)  [unwired: 7 in]
            n4847 = call-dynamic "Write State Machine.vi"("error in (no error)"=w11542, "State Machine.lvclass"=w11554, "Device in"=w11552) -> ("error out"=w11556:errorcluster, "Device out"=w11555:refnum<class "Channel.lvclass">)  [unwired: 7 in]
            n4848 = call-dynamic "Write Channel.vi"("error in (no error)"=w11556, "Channel.lvclass"=w11555, "Acquisition in"=w11526) -> ("error out"=w11521:errorcluster, "Acquisition out"=w11522:refnum<class "Acquisition.lvclass">)  [unwired: 7 in]
          }
        }
        n4849 = case shown="True" w11314 {
          tunnel: [w11557 w11591] -> w11298
          tunnel: [w11558 w11590] -> w11299
          tunnel: w11316 -> [w11558 w11561]
          tunnel: w11315 -> [w11557 w11560]
          tunnel: w11288 -> [_ w11559]
          frame False {
          }
          frame True {
            # "nome do arquivo .cfg"
            # "seção no arquivo .cfg"
            n4850 = call-dynamic "Read Channel.vi"("error in (no error)"=w11560, "Acquisition in"=w11561) -> ("error out"=w11592:errorcluster, "Channel.lvclass"=w11593:refnum<class "Channel.lvclass">, "Acquisition out"=w11594:refnum<class "Acquisition.lvclass">)  [unwired: 7 in]
            n4851 = call-dynamic "Read Interface.vi"("error in (no error)"=w11592, "Channel in"=w11593) -> ("error out"=w11583:errorcluster, "Interface.lvclass"=w11582:refnum<class "Interface.lvclass">, "Channel out"=w11595:refnum<class "Channel.lvclass">)  [unwired: 7 in]
            n4852 = call-dynamic "Get CCD_Config.vi"("error in (no error)"=w11583, "Interface in"=w11582) -> ("error out"=w11585:errorcluster, "output cluster"=w11586:T31, "Interface out"=w11581:refnum<class "Interface.lvclass">)  [unwired: 7 in]
            n4853 = Bundle By Name(cluster=w11586, "TRIGGER_MODE"=w11559) -> (w11584:T31)
            n4854 = call-dynamic "Set CCD_Config.vi"("error in (no error)"=w11585, "input cluster"=w11584, "Interface in"=w11581) -> ("error out"=w11587:errorcluster, "Interface out"=w11580:refnum<class "Interface.lvclass">)  [unwired: 7 in]
            n4855 = Flatten To String(anything=w11584, error in (no error)=w11587) -> (data string=w11589:string, error out=w11588:errorcluster)  [unwired: 2 in, 1 out]
            n4856 = call "Write flatted cluster.vi"("error in (no error)"=w11588, "flatted cluster"=w11589, "Interface in"=w11580) -> ("error out"=w11578:errorcluster, "Interface out"=w11579:refnum<class "Interface.lvclass">)  [unwired: 7 in]
